vi "Sub Routing program.vi"(0 "queue Out in":refnum<queue>, 2 "Table":refnum<vi>, 3 "Feature Step Enable":T1(array[cluster]), 5 "error in (no error)":errorcluster, 7 "Tracibility":bool, 8 "FeedBack Channel":string[](array[string]), 9 "Test Name":refnum<vi>, 10 "Image":refnum<vi>) -> (14 "Queue out":refnum<queue>, 16 "reference out":refnum<vi>, 17 "Error":bool, 19 "error out":errorcluster)   [LabVIEW 2015]
uses:
  Test  enqueue/AutoTest seq.ctl
  Galobal variable_TI.vi
panel:
  out "2D Picture 2":picture
  out "error out 2":errorcluster
  out "2D Picture":picture
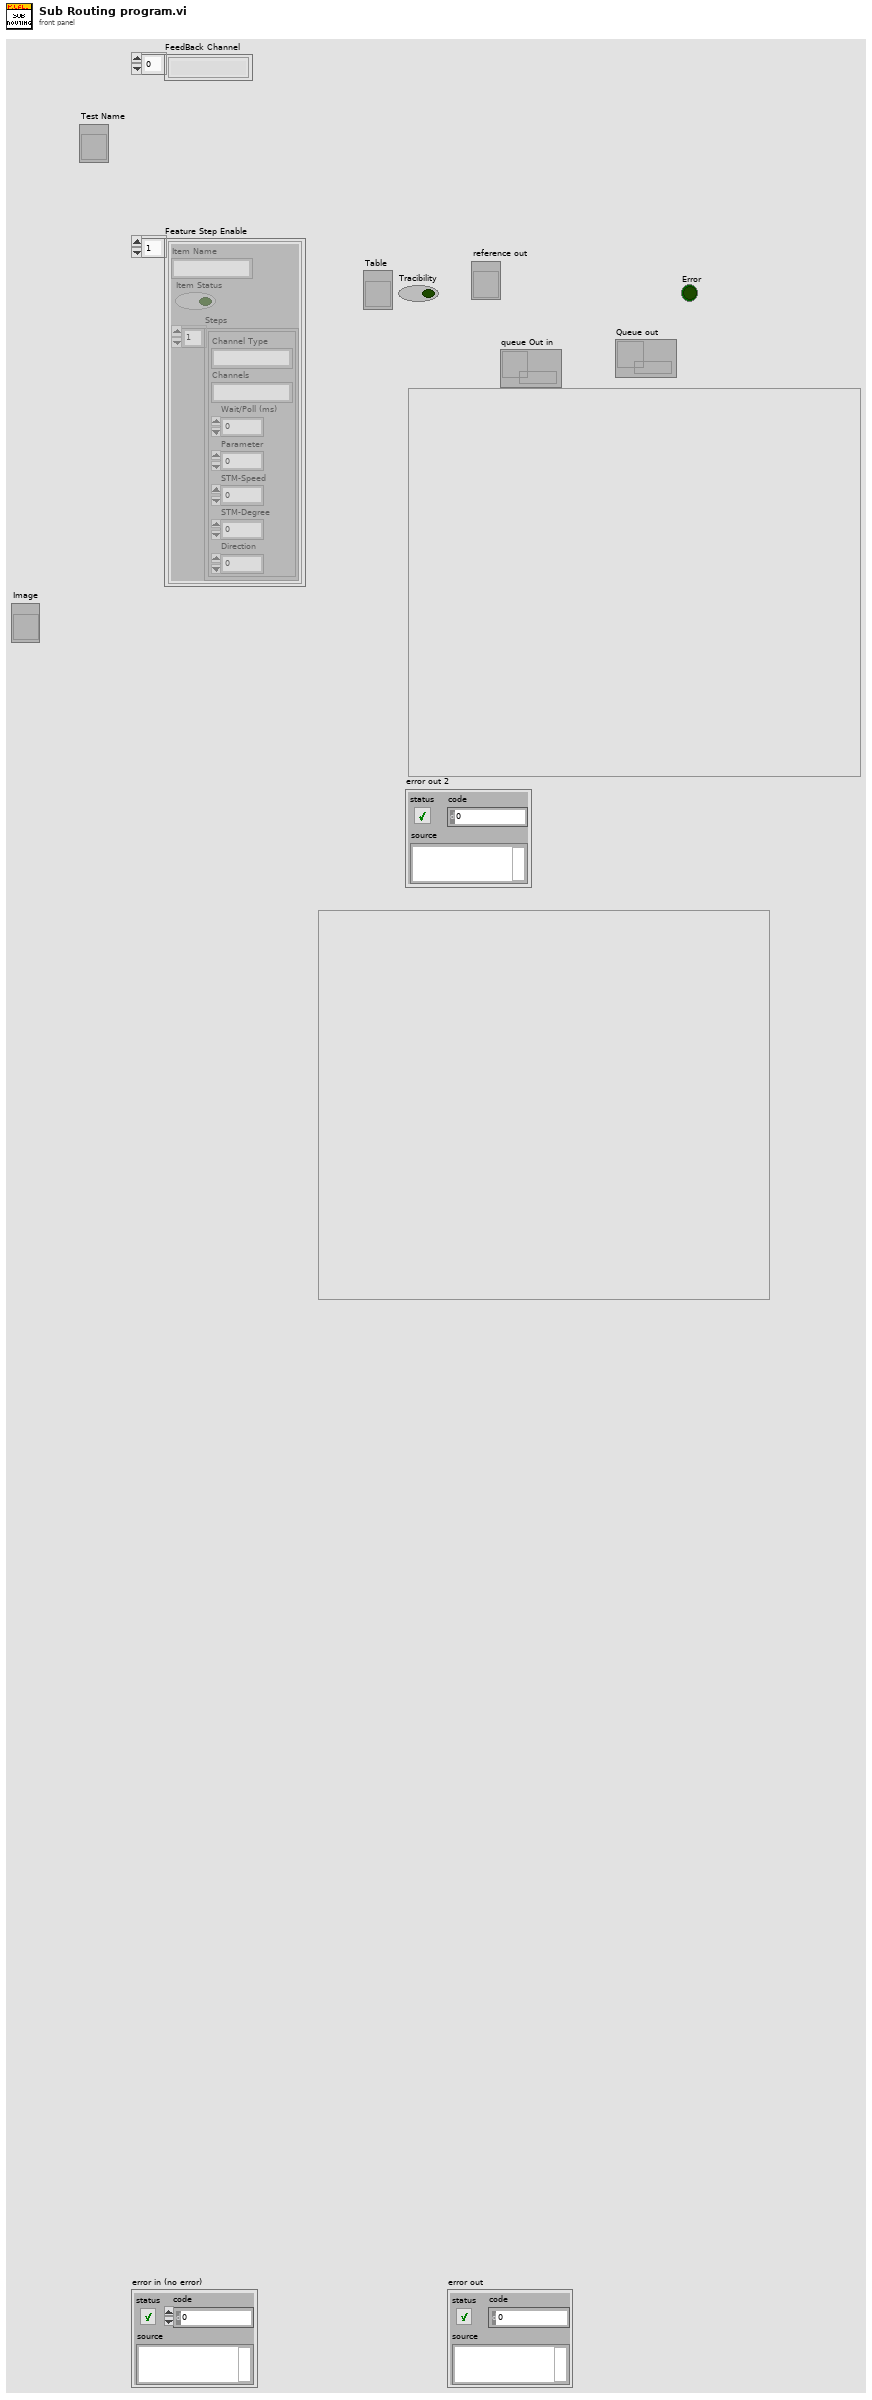
[diagram p1: front panel]
types:
  T1 = cluster{"Item Name":string, "Item Status":bool, "Steps":cluster{"Channel Type":string, "Channels":string, "Wait/Poll (ms)":u32, "Parameter":u8, "STM-Speed":i32, "STM-Degree":u32, "Direction":u8}[]}[]
  T2 = cluster{"Zoom Factor":sgl, "Horizontal position":sgl, "Vertical position":sgl}[]
  T3 = cluster{"Channel Type":string, "Channels":string, "Wait/Poll (ms)":u32, "Parameter":u8, "STM-Speed":i32, "STM-Degree":u32, "Direction":u8}[]
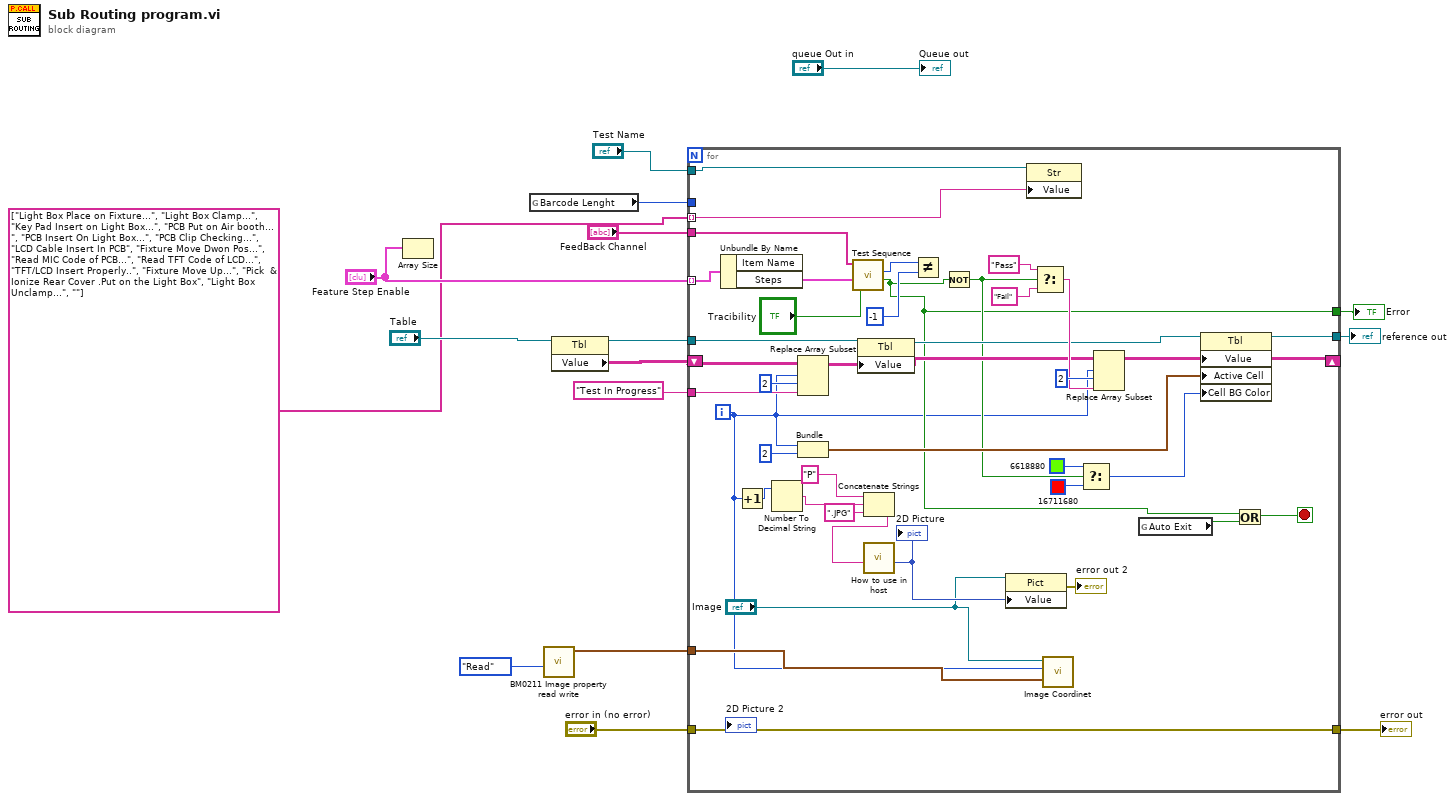
[diagram p0: block diagram]
diagram:
  n1 = Array Size(array="Feature Step Enable") -> ()  [unwired: 1 out]
  n2 = global read "Galobal variable_TI.vi" "Barcode Lenght"() -> (w15:i32)
  n3 = call "BM0211 Image property read write.vi"("Read write"=enum16{"write", "Read"}."Read") -> ("Out"=w2:T2)  [unwired: 9 in, 1 out]
  n4 = property class="Tbl"(reference="Table") -> (reference out=w9:refnum<vi>, "Value"=w12:string[][])  [unwired: 1 in, 1 out]
  n5 = for {
    tunnel: "Feature Step Enable" -> [w56] mode=indexing
    tunnel: "FeedBack Channel" -> [w53]
    tunnel: w15 -> [_]
    shift-right: [w37] -> _
    shift-left: w12 -> [w49]
    tunnel: "Test In Progress" ("new element/subarray") -> [w48]
    tunnel: w9 -> [w47]
    tunnel: [w38] -> w8
    tunnel: "error in (no error)" -> [w36]
    tunnel: [w36] -> w6
    tunnel: [w31] -> w5
    tunnel: "Test Name" -> [w30]
    tunnel: w2 -> [w22]
    tunnel: string[] ["Light Box Place on Fixture...", "Light Box Clamp...", "Key Pad Insert on Light Box...", "PCB Put on Air booth...", "PCB Insert On Light Box...", "PCB Clip Checking...", "LCD Cable Insert In PCB", "Fixture Move Dwon Pos...", "Read MIC Code of PCB...", "Read TFT Code of LCD...", "TFT/LCD Insert Properly..", "Fixture Move Up...", "Pick  &  Ionize Rear Cover .Put on the Light Box", "Light Box Unclamp...", ""] -> [w17] mode=indexing
    i -> [w21]
    stop <- w19 stop-if-true
    n6 = Unbundle By Name(w56) -> ("Steps"=w52:T3)  [unwired: 1 out]
    n7 = Increment(x=w21) -> (x+1=w27:i32)
    n8 = Number To Decimal String(number=w27) -> (decimal integer string=w25:string)  [unwired: 1 in]
    n9 = Replace Array Subset(array=w49, new element=w48, index (row)=w21, index (col)=2 ("disabled index (col)")) -> (w44:string[][])
    n10 = Bundle(w21, 2) -> (w43:cluster{i32, i32})  [unwired: 1 in]
    n11 = call "Test Sequence.vi"("FeedBack Channel"=w53, "Steps"=w52, "Tracibility"="Tracibility") -> ("Out"=w35:i32, "Condition"=w31:bool)  [unwired: 4 in, 1 out]
    n12 = property class="Tbl"(reference=w47, "Value"=w44) -> (reference out=w39:refnum<vi>)  [unwired: 1 in, 1 out]
    n13 = Concatenate Strings("P" ("string"), w25, ".JPG" ("string")) -> (w24:string)
    n14 = call "How to use in host.vi"("element"=w24) -> ("2D Picture"=w29:picture)  [unwired: 9 in, 1 out]
    "2D Picture" <- w29
    n15 = Not Equal?(x=w35, y=-1) -> ()  [unwired: 1 out]
    n16 = Not(x=w31) -> (.not. x?=w32:bool)
    n17 = property class="Pict"(reference="Image", "Value"=w29) -> (error out=→"error out 2":errorcluster)  [unwired: 1 in, 1 out]
    n18 = property class="Str"(reference=w30, "Value"=w17) -> ()  [unwired: 1 in, 2 out]
    n19 = Select(t="Pass", s=w32, f="Fail") -> (s? t:f=w45:string)
    n20 = call "Image Coordinet.vi"("Out"=w22, "index of element"=w21, "Picture in"="Image") -> ()  [unwired: 9 in]
    n21 = Select(t=u32 6618880 ("Color Box"), s=w32, f=u32 16711680 ("Color Box")) -> (s? t:f=w40:u32)
    n22 = Replace Array Subset(array=w44, new element=w45, index (row)=w21, index (col)=2 ("disabled index (col)")) -> (w37:string[][])
    n23 = global read "Galobal variable_TI.vi" "Auto Exit"() -> (w33:bool)
    n24 = property class="Tbl"(reference=w39, "Value"=w37, "Active Cell"=w43, "Cell BG Color"=w40) -> (reference out=w38:refnum<vi>)  [unwired: 1 in, 1 out]
    n25 = Or(x=w31, y=w33) -> (x .or. y?=w19:bool)
  }
  "error out" <- w6
  "reference out" <- w8
  "Error" <- w5
  "Queue out" <- "queue Out in"
